vi "Auton - Drive Forward.vi"(11 "Auton States":T1=enum."Drive Forward") -> ()   [LabVIEW 2016]
uses:
  Auton - Drive Forward States.ctl
panel:
  in  "Drive Forward SP":dbl=72.0
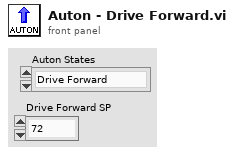
[diagram p1: front panel]
types:
  T1 = typedef "Auton - Drive Forward States.ctl" = enum16{"Stop", "Reset Encoders", "Drive Forward"}
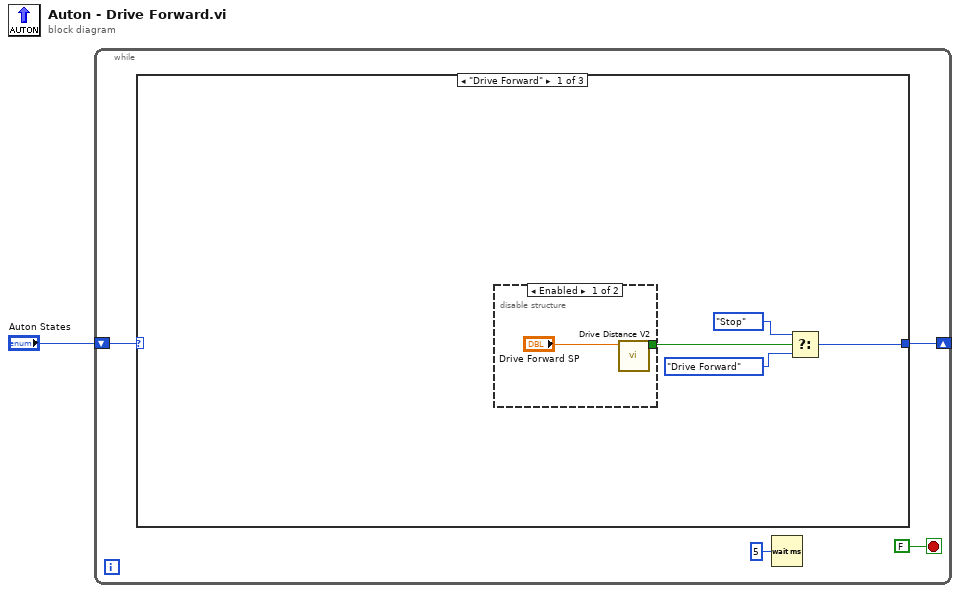
[diagram p0: block diagram]
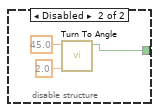
[diagram p2: hidden frame]
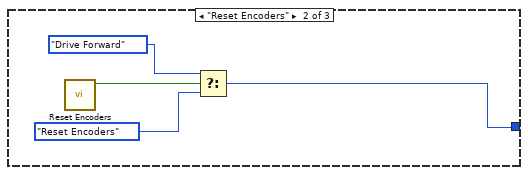
[diagram p3: hidden frame]
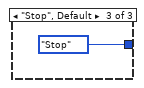
[diagram p4: hidden frame]
diagram:
  n1 = while {
    shift-right: [w3] -> _
    shift-left: "Auton States" -> [w4]
    stop <- FALSE stop-if-true
    n2 = case shown="\"Drive Forward\"" w4 {
      tunnel: [w9 w16 Auton_-_Drive_Forward_States."Stop" ("Auton States")] -> w3
      frame "Drive Forward" {
        n3 = disable-structure shown="Enabled" {
          disable-tunnel: [w11 w12] -> w6
          frame Enabled {
            n4 = call "Drive Distance V2.vi"("Distance Set Point"="Drive Forward SP") -> ("Done?"=w11:bool)  [unwired: 10 in]
          }
          frame Disabled {
            n5 = call "Turn To Angle.vi"("Turn Angle Tolerance"=2.0, "Setpoint"=45.0) -> ("Done?"=w12:bool)  [unwired: 9 in]
          }
        }
        n6 = Select(t=Auton_-_Drive_Forward_States."Stop" ("Auton States"), s=w6, f=Auton_-_Drive_Forward_States."Drive Forward") -> (s? t:f=w9:T1)
      }
      frame "Reset Encoders" {
        n7 = call "Reset Encoders.vi"() -> ("Done?"=w18:bool)  [unwired: 11 in]
        n8 = Select(t=Auton_-_Drive_Forward_States."Drive Forward" ("Auton States"), s=w18, f=Auton_-_Drive_Forward_States."Reset Encoders") -> (s? t:f=w16:T1)
      }
      frame "Stop", Default {
      }
    }
    n9 = Wait (ms)(milliseconds to wait=u32 5) -> ()  [unwired: 1 out]
  }
